vi "edittest write test steps to file.vi"(8 "error in (no error)":errorcluster, 10 "Sequence Steps":T1[](array[typedef]), 11 "File Refnum In":T2) -> (0 "error out":errorcluster, 3 "File Refnum Out":T2)   [LabVIEW 2011]
uses:
  <vilib>/Utility/config.llb/Config Data RefNum.ctl
  server/database/Steps/Step Record.ctl
  <vilib>/Utility/config.llb/Write Key (I32).vi
  <vilib>/Utility/config.llb/Write Key (String).vi
  <vilib>/Utility/config.llb/NI_LVConfig.lvlib
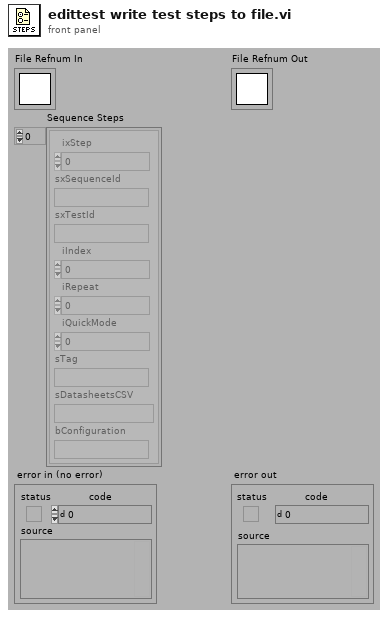
[diagram p1: front panel]
types:
  T1 = typedef "Step Record.ctl" = cluster{"ixStep":i32, "sxSequenceId":string, "sxTestId":string, "iIndex":i32, "iRepeat":i32, "iQuickMode":i32, "sTag":string, "sDatasheetsCSV":string, "bConfiguration":string}
  T2 = typedef "NI_LVConfig.lvlib/Config Data RefNum.ctl" = refnum<k1>
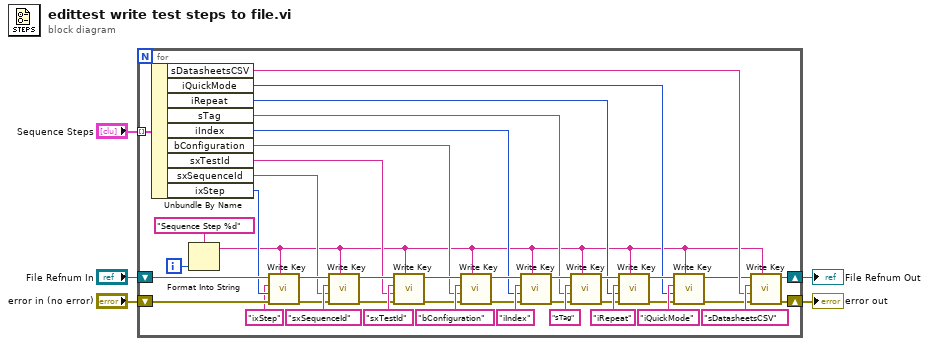
[diagram p0: block diagram]
diagram:
  n1 = for {
    shift-right: [w7] -> w4
    shift-left: "File Refnum In" -> [w43]
    shift-right: [w6] -> w5
    shift-left: "error in (no error)" -> [w44]
    tunnel: "Sequence Steps" -> [w45] mode=indexing
    i -> [w46]
    n2 = Unbundle By Name(w45) -> ("sDatasheetsCSV"=w10:string, "iQuickMode"=w13:i32, "iRepeat"=w14:i32, "sTag"=w15:string, "iIndex"=w16:i32, "bConfiguration"=w17:string, "sxTestId"=w18:string, "sxSequenceId"=w19:string, "ixStep"=w42:i32)
    n3 = Format Into String(format string="Sequence Step %d", w46) -> (resulting string=w8:string)  [unwired: 2 in, 1 out]
    n4 = call-poly <vilib>:"Write Key.vi"("section"=w8, "error in (no error)"=w44, "value"=w42, "key"="ixStep", "refnum"=w43) -> ("error out"=w34:errorcluster, "refnum out"=w25:T2)  [unwired: 5 out]
    n5 = call-poly <vilib>:"Write Key.vi"("section"=w8, "error in (no error)"=w34, "value"=w19, "key"="sxSequenceId", "refnum"=w25) -> ("error out"=w33:errorcluster, "refnum out"=w26:T2)  [unwired: 1 in, 4 out]
    n6 = call-poly <vilib>:"Write Key.vi"("section"=w8, "error in (no error)"=w33, "value"=w18, "key"="sxTestId", "refnum"=w26) -> ("error out"=w20:errorcluster, "refnum out"=w21:T2)  [unwired: 1 in, 4 out]
    n7 = call-poly <vilib>:"Write Key.vi"("section"=w8, "error in (no error)"=w20, "value"=w17, "key"="bConfiguration", "refnum"=w21) -> ("error out"=w23:errorcluster, "refnum out"=w22:T2)  [unwired: 1 in, 4 out]
    n8 = call-poly <vilib>:"Write Key.vi"("section"=w8, "error in (no error)"=w23, "value"=w16, "key"="iIndex", "refnum"=w22) -> ("error out"=w32:errorcluster, "refnum out"=w27:T2)  [unwired: 5 out]
    n9 = call-poly <vilib>:"Write Key.vi"("section"=w8, "error in (no error)"=w32, "value"=w15, "key"="sTag", "refnum"=w27) -> ("error out"=w31:errorcluster, "refnum out"=w28:T2)  [unwired: 1 in, 4 out]
    n10 = call-poly <vilib>:"Write Key.vi"("section"=w8, "error in (no error)"=w31, "value"=w14, "key"="iRepeat", "refnum"=w28) -> ("error out"=w30:errorcluster, "refnum out"=w29:T2)  [unwired: 5 out]
    n11 = call-poly <vilib>:"Write Key.vi"("section"=w8, "error in (no error)"=w30, "value"=w13, "key"="iQuickMode", "refnum"=w29) -> ("error out"=w11:errorcluster, "refnum out"=w9:T2)  [unwired: 5 out]
    n12 = call-poly <vilib>:"Write Key.vi"("section"=w8, "error in (no error)"=w11, "value"=w10, "key"="sDatasheetsCSV", "refnum"=w9) -> ("error out"=w6:errorcluster, "refnum out"=w7:T2)  [unwired: 1 in, 4 out]
  }
  "error out" <- w5
  "File Refnum Out" <- w4
